vi "EN50160 Aggregation 3sec.vi"(0 "signaling voltage RMS values":dbl[](array[numeric]), 4 "system info in":refnum<class "EP System Info.lvclass">, 5 "error in (no error)":errorcluster, 6 "reset? (F)":bool, 7 "voltage flags? (F)":bool[](array[boolean]), 8 "data timestamp":timestamp) -> (14 "3s values":T1, 18 "system info out":refnum<class "EP System Info.lvclass">, 19 "error out":errorcluster)   [LabVIEW 2014, in "NI_EP_Power Quality.lvlib"]
doc: "Calculates aggregated values of power quality parameters for specific intervals. You use the aggregated values for further evaluations according to EN 50160:2007. The aggregation methods are compliant with Class S in IEC 61000-4-30:2008. The aggregation is based on a 10-cycle time interval for a 50 Hz power system or 12-cycle time interval for a 60 Hz power system. There is no overlap between aggregation intervals. This VI automatically restarts accumulation at the beginning of the next 10/12-cycle time interval after the previous interval expires. You must manually select the polymorphic instance you want to use.\n\nThis VI supports measuring single-bus single-line or multiple-bus single-line systems."
uses:
  <vilib>/addons/Electrical Power/PQ/NI_EP_Power Quality.lvlib
  <vilib>/addons/Electrical Power/PQ/Common/Classes/System Info/EP System Info.lvclass
  <vilib>/addons/Electrical Power/PQ/Common/Controls/ep_Aggregation Settings.ctl
  <vilib>/addons/Electrical Power/PQ/Aggregation/Custom Aggregation (1D DBL Array).vi
  <vilib>/addons/Electrical Power/PQ/Aggregation/Custom Aggregation (Flags).vi
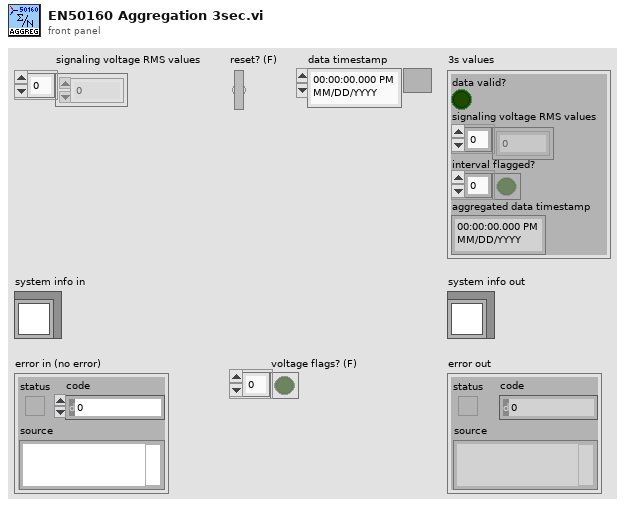
[diagram p1: front panel]
types:
  T1 = cluster{"data valid?":bool, "signaling voltage RMS values":dbl[], "interval flagged?":bool[], "aggregated data timestamp":timestamp}
  T2 = typedef "NI_EP_Power Quality.lvlib/ep_Aggregation Settings.ctl" = cluster{"interval":u32, "interval unit":enum16{"Runs", "Seconds", "Minutes", "Hours", "Days", "Weeks"}, "synchronization of intervals":enum16{"Not synchronized", "Interval rounded"}, "algorithm":enum16{"Average", "RMS"}}
  T3 = cluster{"aggregated data valid?":bool, "aggregated averaged/RMS values":dbl[], "aggregated voltage flags":bool[], "aggregated data timestamp":timestamp}
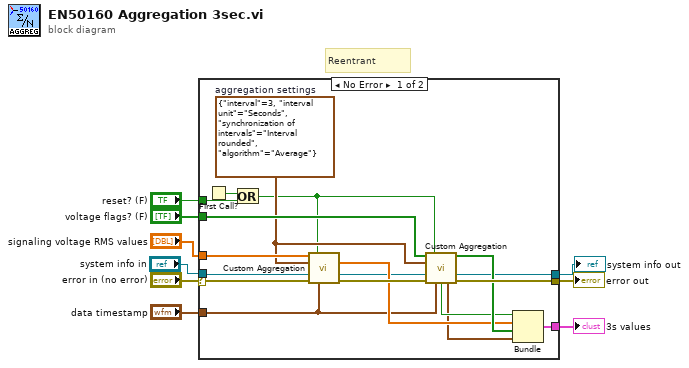
[diagram p0: block diagram]
diagram:
  # "Reentrant"
  n1 = case shown="No Error" "error in (no error)" {
    selector: "error in (no error)" -> [w19 w29]
    tunnel: [w27 _] -> w9
    tunnel: "reset? (F)" -> [w17 _]
    tunnel: [w25 w29] -> w7
    tunnel: "signaling voltage RMS values" -> [w24 _]
    tunnel: "data timestamp" -> [w15 _]
    tunnel: "voltage flags? (F)" -> [w21 _]
    tunnel: "system info in" -> [w14 w28]
    tunnel: [w12 w28] -> w1
    frame No Error {
      w20 = T2 {"interval"=3, "interval unit"=enum."Seconds", "synchronization of intervals"=enum."Interval rounded", "algorithm"=enum."Average"}  # aggregation settings
      n2 = First Call?() -> (First Call?: T/F=w18:bool)
      n3 = Or(x=w18, y=w17) -> (x .or. y?=w16:bool)
      n4 = call-poly <vilib>:"Custom Aggregation.vi"("data in"=w24, "reset? (F)"=w16, "aggregation settings"=w20, "system info in"=w14, "error in (no error)"=w19, "data timestamp"=w15) -> ("aggregated averaged/RMS values"=w22:dbl[], "system info out"=w13:refnum<class "EP System Info.lvclass">, "error out"=w26:errorcluster)  [unwired: 3 in, 4 out]
      n5 = call-poly <vilib>:"Custom Aggregation.vi"("voltage flags? (F)"=w21, "reset? (F)"=w16, "aggregation settings"=w20, "system info in"=w13, "error in (no error)"=w26, "data timestamp"=w15) -> ("aggregated voltage flags"=w23:bool[], "system info out"=w12:refnum<class "EP System Info.lvclass">, "aggregated data valid?"=w11:bool, "aggregated data timestamp"=w10:timestamp, "error out"=w25:errorcluster)  [unwired: 5 in]
      n6 = Bundle("aggregated data valid?"=w11, "aggregated averaged/RMS values"=w22, "aggregated voltage flags"=w23, "aggregated data timestamp"=w10) -> (w27:T3)  [unwired: 1 in]
    }
    frame Error {
    }
  }
  "error out" <- w7
  "3s values" <- w9
  "system info out" <- w1
